vi "GetDisplayName3.vi"(0 "XRef":T10, 1 "State In":T3) -> (14 "Type Name":T2, 15 "Instance Name":T2, 16 "Fatal Error Out":T1)   [LabVIEW 2020, in "Parallel Diagram Block.xnode"]
uses:
  Parallel Diagram Block.xnode
  <vilib>/XNodeSupport/XNodeXNodeRef.ctl
  State.ctl
  Parallel Block/Type Descriptor.ctl
  Parallel Block/Direction.ctl
  Parallel Block/Value Type.ctl
  Parallel Block/Terminal Mode.ctl
  Parallel Block/Terminal Type.ctl
  <vilib>/picture/picture.llb/imagedata.ctl
  <vilib>/XNodeSupport/XNodeString.ctl
  <vilib>/XNodeSupport/XNodeErrorCluster.ctl
  <vilib>/XNodeSupport/NI_XNodeSupport.lvlib
  Parallel Block/Parallel Block.lvlib
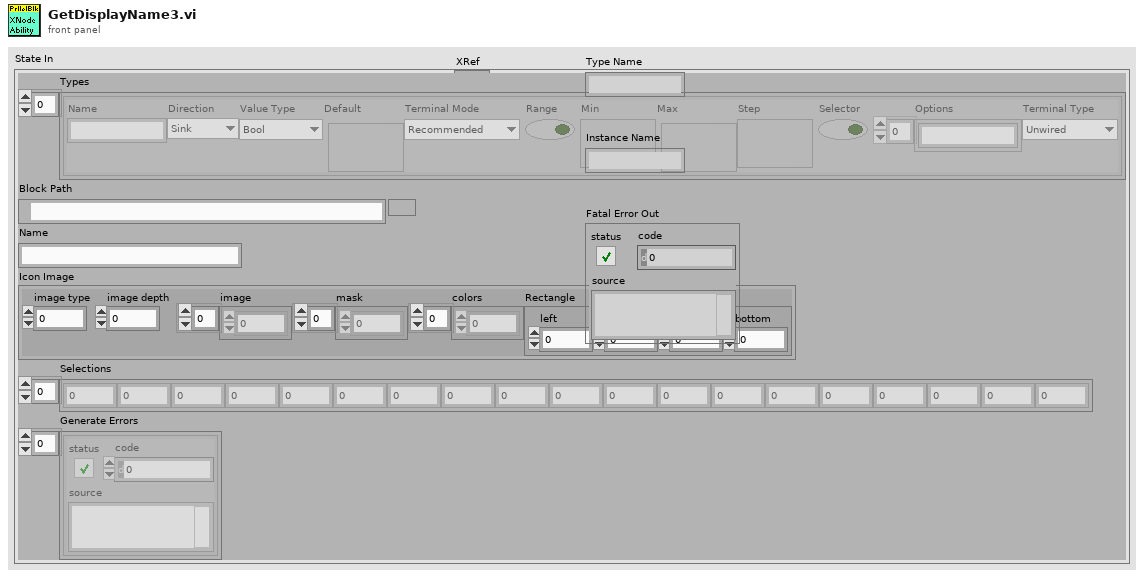
[diagram p1: front panel]
types:
  T1 = typedef "NI_XNodeSupport.lvlib/XNodeErrorCluster.ctl" = errorcluster
  T2 = typedef "NI_XNodeSupport.lvlib/XNodeString.ctl" = string
  T3 = typedef "Parallel Diagram Block.xnode/State.ctl" = cluster{"Types":T4[], "Block Path":path, "Name":string, "Icon Image":T9, "Selections":i32[], "Generate Errors":errorcluster[]}
  T4 = typedef "Parallel Block.lvlib/Type Descriptor.ctl" = cluster{"Name":string, "Direction":T5, "Value Type":T6, "Default":variant, "Terminal Mode":T7, "Range":bool, "Min":variant, "Max":variant, "Step":variant, "Selector":bool, "Options":string[], "Terminal Type":T8}
  T5 = typedef "Parallel Block.lvlib/Direction.ctl" = enum16{"Sink", "Source"}
  T6 = typedef "Parallel Block.lvlib/Value Type.ctl" = enum16{"Unknown", "Bool", "U8", "U16", "U32", "U64", "I8", "I16", "I32", "I64", "SGL", "DBL", "CSG", "CDB", "CDBWfm", "String", "DBLWfm"}
  T7 = typedef "Parallel Block.lvlib/Terminal Mode.ctl" = enum16{"Recommended", "Required", "None"}
  T8 = typedef "Parallel Block.lvlib/Terminal Type.ctl" = enum16{"Unwired", "Connection", "Value", "Control Ref"}
  T9 = typedef "imagedata.ctl" = cluster{"image type":i32, "image depth":i32, "image":u8[], "mask":u8[], "colors":u32[], "Rectangle":cluster{"left":i16, "top":i16, "right":i16, "bottom":i16}}
  T10 = typedef "NI_XNodeSupport.lvlib/XNodeXNodeRef.ctl" = refnum<vi>
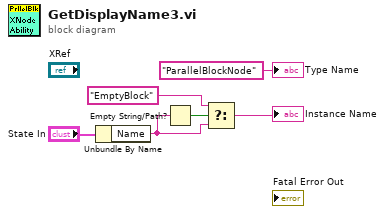
[diagram p0: block diagram]
diagram:
  n1 = Unbundle By Name("State In") -> ("Name"=w3:string)
  n2 = Empty String/Path?(string/path=w3) -> (empty?=w4:bool)
  n3 = Select(t="EmptyBlock", s=w4, f=w3) -> (s? t:f=→"Instance Name":string)
  "Type Name" <- T2 "ParallelBlockNode" ("Type Name")
